vi "Module BL Script.vi"(10 "Scan Direction":u32(ring)=3 items=["Left to Right", "Right to Left", "Top to Bottom", "Bottom to Top"], 11 "Scan Direction L/R":u32(ring) items=["Left to Right", "Right to Left", "Top to Bottom", "Bottom to Top"]) -> (2 "In Range?":bool, 3 "Vertical vector":dbl[](array[numeric]))   [LabVIEW 2011]
uses:
  <vilib>/vision/driver/NI_Vision_Acquisition_Software.lvlib
  <vilib>/vision/NI_Vision_Development_Module.lvlib
panel:
  out "error out":errorcluster
  out "Y":sgl
  out "X":sgl
  out "X Coordinate Pixels":dbl
  out "Y Coordinate Pixels":sgl
  out "Angle Between Lines":dbl
  out "Image Out":T1(plugin-control)
  out "Line Coordinates (calibrated) (Straight Edge (Rake) 2)":T2 {"Point2"."Y" format="%.2f"; "Point2"."X" format="%.2f"; "Point1"."Y" format="%.2f"; "Point1"."X" format="%.2f"}
  out "Edge Coordinates (calibrated) (Straight Edge (Rake) 2)":cluster{"X":sgl, "Y":sgl}[](array[cluster]) {"Y" format="%.2f"; "X" format="%.2f"}
  out "Line Coordinates (calibrated) (Straight Edge (Rake) 1)":T2 {"Point2"."Y" format="%.2f"; "Point2"."X" format="%.2f"; "Point1"."Y" format="%.2f"; "Point1"."X" format="%.2f"}
  out "Edge Coordinates (calibrated) (Straight Edge (Rake) 1)":cluster{"X":sgl, "Y":sgl}[](array[cluster]) {"Y" format="%.2f"; "X" format="%.2f"}
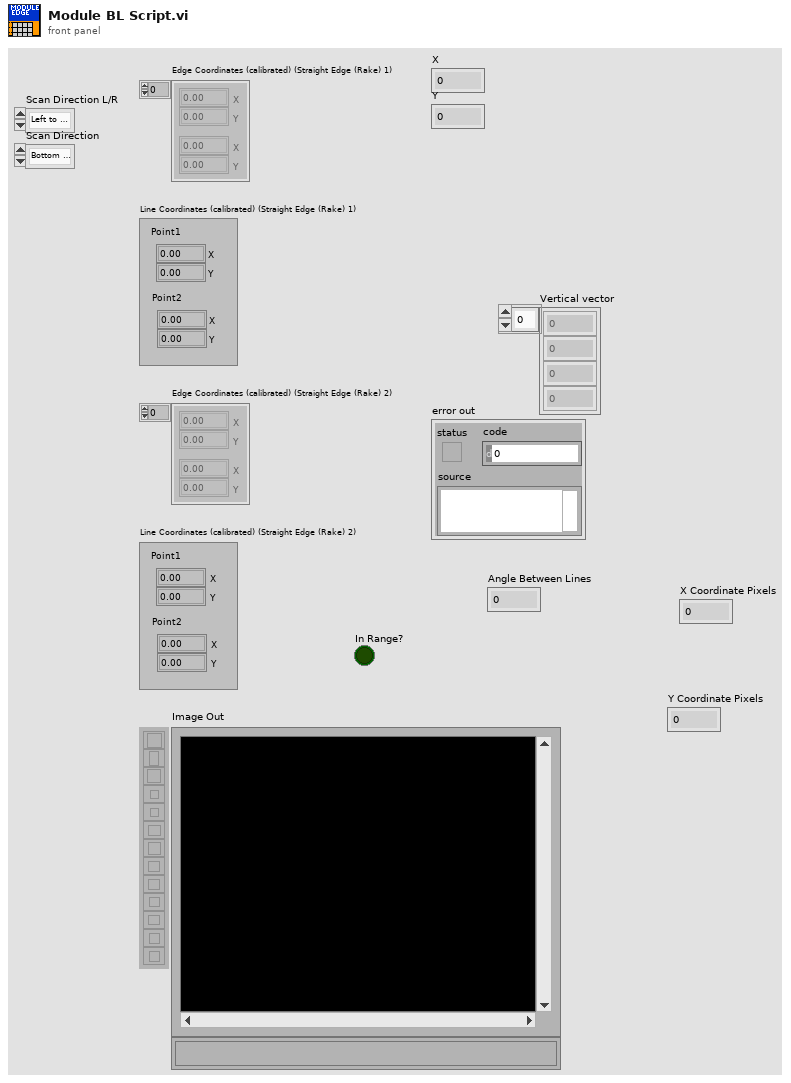
[diagram p1: front panel]
types:
  T1 = typedef "IMAQ Image.ctl" = refnum<image>
  T2 = cluster{"Point1":cluster{"X":sgl, "Y":sgl}, "Point2":cluster{"X":sgl, "Y":sgl}}
  T3 = cluster{"Global Rectangle":i32[], "Contours":cluster{"ID":enum32{"External", "Internal"}, "Type":u32, "Coordinates":i32[]}[]}
  T4 = typedef "IMAQdx.ctl" = refnum<k21>
  T5 = cluster{"Contrast":i32, "Filter width":i32, "Steepness":i32, "Subsampling Ratio":u32, "Scan Direction L/R":u32, "Show Search Area":bool, "Show Search Lines":bool, "Show Edges Found":bool, "Show Result":bool}
  T6 = typedef "IMAQ Rectangle" = cluster{"Left":i32, "Top":i32, "Right":i32, "Bottom":i32, "Rotation":dbl}
  T7 = cluster{"Contrast":i32, "Filter width":i32, "Steepness":i32, "Subsampling Ratio":u32, "Scan Direction":u32, "Show Search Area":bool, "Show Search Lines":bool, "Show Edges Found":bool, "Show Result":bool}
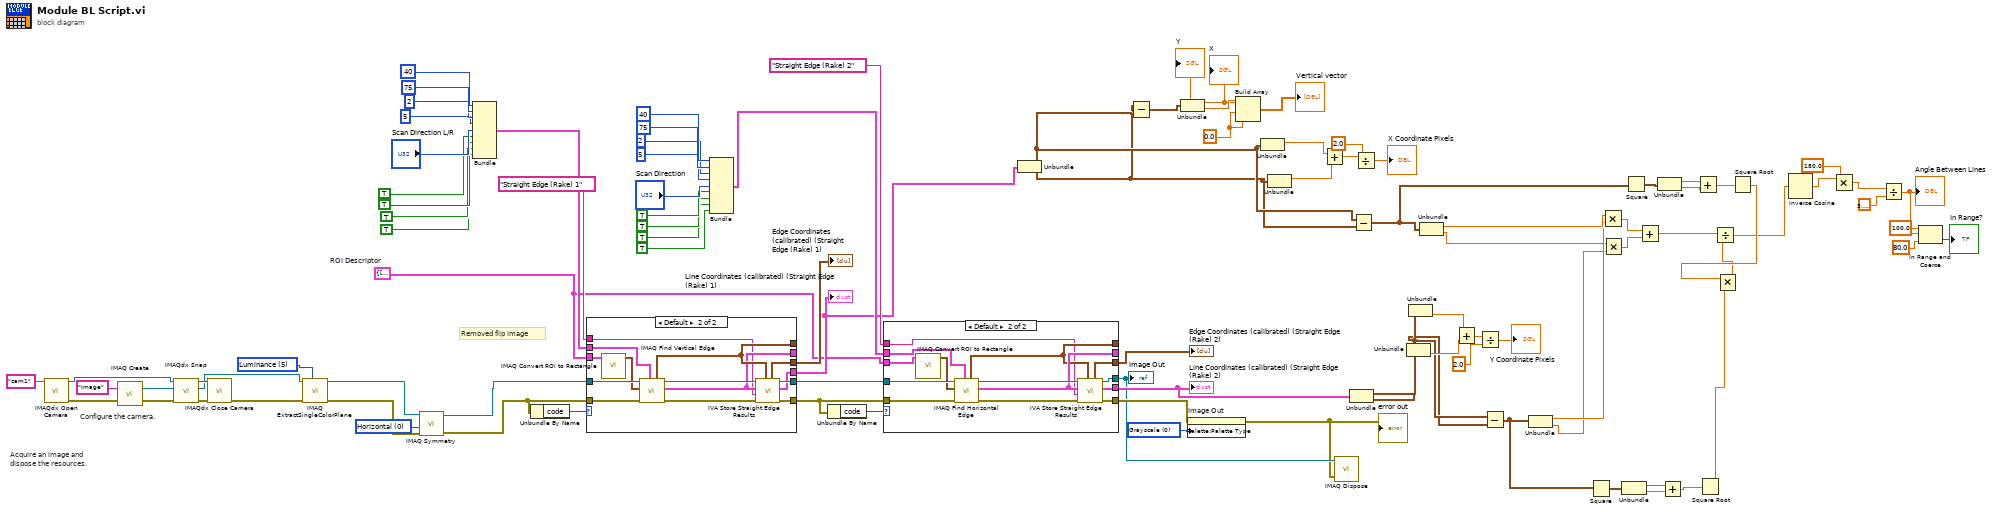
[diagram p0: block diagram]
diagram:
  w1 = u32 0 items=["Horizontal", "Vertical", "Central", "1st Diagonal", "2nd Diagonal"] ("Type of Symmetry")
  w57 = 0.0
  w79 = u32 0 items=["Grayscale", "Binary", "Gradient", "Rainbow", "Temperature", "User Defined"] ("Palette")
  w6 = T3 {"Global Rectangle"=[0, 0, 2650, 1920], "Contours"=[{"ID"=enum."External", "Type"=3, "Coordinates"=[0, 0, 2650, 1920, 0]}]}  # ROI Descriptor
  w90 = 5 items=["Red", "Green", "Blue", "Hue", "Saturation", "Luminance", "Value", "Intensity"] ("Color Plane")
  # "Removed flip image"
  # "Acquire an image and\ndispose the resources."
  # "Configure the camera."
  n1 = call <vilib>:"IMAQdx Open Camera.vi"("Session In"="cam1" ("Interface Name")) -> ("error out"=w97:errorcluster, "Session Out"=w91:T4)  [unwired: 9 in]
  n2 = call "IMAQ Create"("Image Name"="Image", "error in (no error)"=w97) -> ("New Image"=w93:T1, "error out"=w92:errorcluster)  [unwired: 3 in]
  n3 = call <vilib>:"IMAQdx Snap.vi"("error in"=w92, "Image In"=w93, "Session In"=w91) -> ("error out"=w95:errorcluster, "Image Out"=w89:T1, "Session Out"=w96:T4)  [unwired: 6 in]
  n4 = call <vilib>:"IMAQdx Close Camera.vi"("error in"=w95, "Session In"=w96) -> ("error out"=w94:errorcluster)  [unwired: 9 in]
  n5 = call "IMAQ ExtractSingleColorPlane"("Color Plane"=w90, "error in (no error)"=w94, "Image Src"=w89) -> ("error out"=w4:errorcluster, "Image Dst Out"=w5:T1)  [unwired: 7 in]
  n6 = call "IMAQ Symmetry"("error in (no error)"=w4, "Type of Symmetry"=w1, "Image Src"=w5) -> ("error out"=w2:errorcluster, "Image Dst Out"=w3:T1)  [unwired: 2 in]
  n7 = Bundle("Contrast"=40, "Filter width"=75, "Steepness"=2, "Subsampling Ratio"=u32 5, "Scan Direction L/R"="Scan Direction L/R", "Show Search Area"=TRUE, "Show Search Lines"=TRUE, "Show Edges Found"=TRUE, "Show Result"=TRUE) -> (w73:T5)  [unwired: 1 in]
  n8 = Unbundle By Name(w2) -> ("code"=w85:i32)
  n9 = case shown="Default" w85 {
    tunnel: w3 -> [w100 w114]
    tunnel: w2 -> [_ w113]
    tunnel: w73 -> [_ w112]
    tunnel: w6 -> [_ w111]
    tunnel: [w100 w108] -> w84
    tunnel: [_ w106] -> w88
    tunnel: [_ w105] -> _
    tunnel: [_ w104] -> w87
    tunnel: [_ w103] -> w58
    tunnel: [_ w102] -> _
    tunnel: "Straight Edge (Rake) 1" ("Step Name") -> [_ w101]
    frame -1074396199, -1074396198 {
      # "Discard Coordinate System Error"
    }
    frame Default {
      n10 = call "IMAQ Convert ROI to Rectangle"("ROI Descriptor"=w111) -> ("Rectangle"=w110:T6)  [unwired: 8 in, 1 out]
      n11 = call "IMAQ Find Vertical Edge"("Settings"=w112, "error in (no error)"=w113, "Rectangle"=w110, "Image"=w114) -> ("error out"=w107:errorcluster, "Line Coordinates"=w102:T2, "Image Out"=w109:T1, "Edge Coordinates"=w105:cluster{"X":sgl, "Y":sgl}[])  [unwired: 2 in, 2 out]
      n12 = call <vilib>:"IVA Store Straight Edge Results.vi"("Edge Coordinates"=w105, "error in (no error)"=w107, "Step Name"=w101, "Line Coordinates"=w102, "Image in"=w109) -> ("error out"=w106:errorcluster, "Line Coordinates (calibrated)"=w103:T2, "Image dup"=w108:T1, "Edge Coordinates (calibrated)"=w104:cluster{"X":sgl, "Y":sgl}[])  [unwired: 3 in]
    }
  }
  "Edge Coordinates (calibrated) (Straight Edge (Rake) 1)" <- w87
  "Line Coordinates (calibrated) (Straight Edge (Rake) 1)" <- w58
  n13 = Bundle("Contrast"=40, "Filter width"=75, "Steepness"=2, "Subsampling Ratio"=u32 5, "Scan Direction"="Scan Direction", "Show Search Area"=TRUE, "Show Search Lines"=TRUE, "Show Edges Found"=TRUE, "Show Result"=TRUE) -> (w61:T7)  [unwired: 1 in]
  n14 = Unbundle By Name(w88) -> ("code"=w80:i32)
  n15 = case shown="Default" w80 {
    tunnel: w61 -> [_ w129]
    tunnel: w84 -> [w115 w128]
    tunnel: w88 -> [_ w127]
    tunnel: w6 -> [_ w126]
    tunnel: [w115 w123] -> w8
    tunnel: [_ w121] -> w83
    tunnel: [_ w120] -> _
    tunnel: [_ w119] -> _
    tunnel: "Straight Edge (Rake) 2" ("Step Name") -> [_ w118]
    tunnel: [_ w117] -> w81
    tunnel: [_ w116] -> w27
    frame -1074396199, -1074396198 {
      # "Discard Coordinate System Error"
    }
    frame Default {
      n16 = call "IMAQ Convert ROI to Rectangle"("ROI Descriptor"=w126) -> ("Rectangle"=w125:T6)  [unwired: 8 in, 1 out]
      n17 = call "IMAQ Find Horizontal Edge"("Settings"=w129, "error in (no error)"=w127, "Rectangle"=w125, "Image"=w128) -> ("error out"=w122:errorcluster, "Line Coordinates"=w120:T2, "Image Out"=w124:T1, "Edge Coordinates"=w119:cluster{"X":sgl, "Y":sgl}[])  [unwired: 2 in, 2 out]
      n18 = call <vilib>:"IVA Store Straight Edge Results.vi"("Edge Coordinates"=w119, "error in (no error)"=w122, "Step Name"=w118, "Line Coordinates"=w120, "Image in"=w124) -> ("error out"=w121:errorcluster, "Line Coordinates (calibrated)"=w116:T2, "Image dup"=w123:T1, "Edge Coordinates (calibrated)"=w117:cluster{"X":sgl, "Y":sgl}[])  [unwired: 3 in]
    }
  }
  "Edge Coordinates (calibrated) (Straight Edge (Rake) 2)" <- w81
  "Line Coordinates (calibrated) (Straight Edge (Rake) 2)" <- w27
  "Image Out" <- w8
  n19 = Unbundle(w58) -> ("Point1"=w18:cluster{"X":sgl, "Y":sgl}, "Point2"=w17:cluster{"X":sgl, "Y":sgl})
  n20 = Subtract(x=w17, y=w18) -> (x-y=w55:cluster{"X":sgl, "Y":sgl})
  n21 = Unbundle(w55) -> ("X"=w53:sgl, "Y"=w54:sgl)
  "X" <- w53
  "Y" <- w54
  n22 = property on="Image Out" class="ImageControl"(error in=w83, "Palette:Palette Type"=w79) -> (error out=w7:errorcluster)  [unwired: 1 in, 1 out]
  "error out" <- w7
  n23 = Build Array(w54, w53, w57, w57) -> (→"Vertical vector":dbl[])
  n24 = Unbundle(w18) -> ("X"=w21:sgl)  [unwired: 1 out]
  n25 = Unbundle(w17) -> ("X"=w20:sgl)  [unwired: 1 out]
  n26 = Add(x=w21, y=w20) -> (x+y=w23:sgl)
  n27 = call "IMAQ Dispose"("Image"=w8, "error in (no error)"=w7) -> ()  [unwired: 4 in, 1 out]
  n28 = Unbundle(w27) -> ("Point1"=w26:cluster{"X":sgl, "Y":sgl}, "Point2"=w25:cluster{"X":sgl, "Y":sgl})
  n29 = Subtract(x=w18, y=w17) -> (x-y=w16:cluster{"X":sgl, "Y":sgl})
  n30 = Divide(x=w23, y=2.0) -> (x/y=→"X Coordinate Pixels":dbl)
  n31 = Unbundle(w25) -> ("Y"=w36:sgl)  [unwired: 1 out]
  n32 = Unbundle(w26) -> ("Y"=w37:sgl)  [unwired: 1 out]
  n33 = Unbundle(w16) -> ("X"=w12:sgl, "Y"=w10:sgl)
  n34 = Add(x=w37, y=w36) -> (x+y=w35:sgl)
  n35 = Divide(x=w35, y=sgl 2.0) -> (x/y=→"Y Coordinate Pixels":sgl)
  n36 = Subtract(x=w26, y=w25) -> (x-y=w28:cluster{"X":sgl, "Y":sgl})
  n37 = Unbundle(w28) -> ("X"=w11:sgl, "Y"=w9:sgl)
  n38 = Square(x=w28) -> (x^2=w32:cluster{"X":sgl, "Y":sgl})
  n39 = Multiply(x=w12, y=w11) -> (x*y=w52:sgl)
  n40 = Multiply(x=w10, y=w9) -> (x*y=w51:sgl)
  n41 = Unbundle(w32) -> ("X"=w31:sgl, "Y"=w30:sgl)
  n42 = Square(x=w16) -> (x^2=w15:cluster{"X":sgl, "Y":sgl})
  n43 = Add(x=w52, y=w51) -> (x+y=w49:sgl)
  n44 = Unbundle(w15) -> ("X"=w14:sgl, "Y"=w13:sgl)
  n45 = Add(x=w31, y=w30) -> (x+y=w29:sgl)
  n46 = Add(x=w14, y=w13) -> (x+y=w50:sgl)
  n47 = Square Root(x=w29) -> (sqrt(x)=w24:sgl)
  n48 = Square Root(x=w50) -> (sqrt(x)=w48:sgl)
  n49 = Multiply(x=w48, y=w24) -> (x*y=w47:sgl)
  n50 = Divide(x=w49, y=w47) -> (x/y=w46:sgl)
  n51 = Inverse Cosine(1:w46) -> (0:w45:sgl)
  n52 = Multiply(x=w45, y=sgl 180.0) -> (x*y=w43:sgl)
  n53 = Divide(x=w43, y=3.141592653589793) -> (x/y=w41:dbl)
  "Angle Between Lines" <- w41
  n54 = In Range and Coerce(upper limit=100.0, x=w41, lower limit=80.0) -> (In Range?=→"In Range?":bool)  [unwired: 1 out]
